vi "Init_Simulator(SubVI).vi"(10 "Enable 3D Visualization":bool, 11 "appended path":path) -> (0 "error out":errorcluster, 1 "robot body ref":refnum<k20>, 2 "starter kit differential steering frame":refnum<class "NI_Robotics_Differential Steering Frame.lvclass">, 3 "NI_Robotics_Starter Kit Host_Sim_2.0 out":refnum<class "NI_Robotics_Starter Kit Host_Sim_2.0.lvclass">, 5 "Current_Position":T1, 7 "map reference out":refnum<data-value>)   [LabVIEW 2017]
uses:
  Ctl/Current_Position.ctl
  <vilib>/robotics/Starter Kit/2.0/Sim Host Interface/NI_Robotics_Starter Kit Host_Sim_2.0.lvclass
  E:/PROGRAM FILES/National Instruments/LabVIEW 2017/vi.lib/robotics/Starter Kit/Host Interface/NI_Robotics_Starter Kit Host.lvclass
  <vilib>/robotics/Steering/Differential Steering Frame/NI_Robotics_Differential Steering Frame.lvclass
  <vilib>/robotics/Navigation/shared/WorldMap/OccupancyGridWorldMap/NI_Robotics_OccupancyGridWorldMap.lvclass
  <vilib>/robotics/Simulator/Interface/Simulator References/Get Robot Body Reference.vi
  GBL/GBL_variables.vi
  <vilib>/robotics/Simulator/NI_Robotics_Simulator.lvlib
  <vilib>/robotics/Starter Kit/2.0/NI_Robotics_Starter Kit Host_2.0.lvlib
  <resource>/objmgr/LVODE.rc
  <vilib>/robotics/Starter Kit/Host Interface/NI_Robotics_Starter Kit Host.lvclass
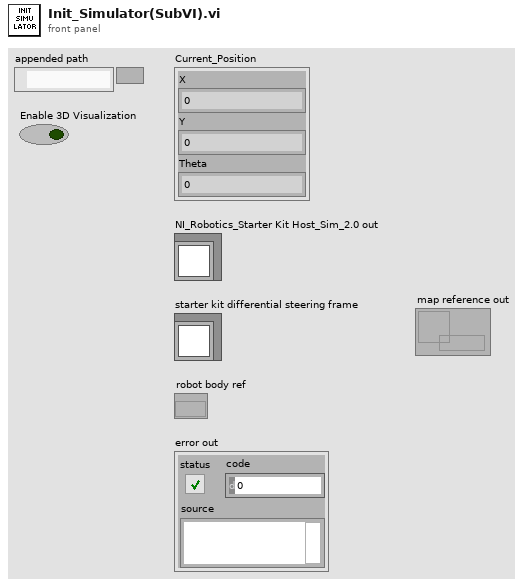
[diagram p1: front panel]
types:
  T1 = typedef "Current_Position.ctl" = cluster{"X":dbl, "Y":dbl, "Theta":dbl}
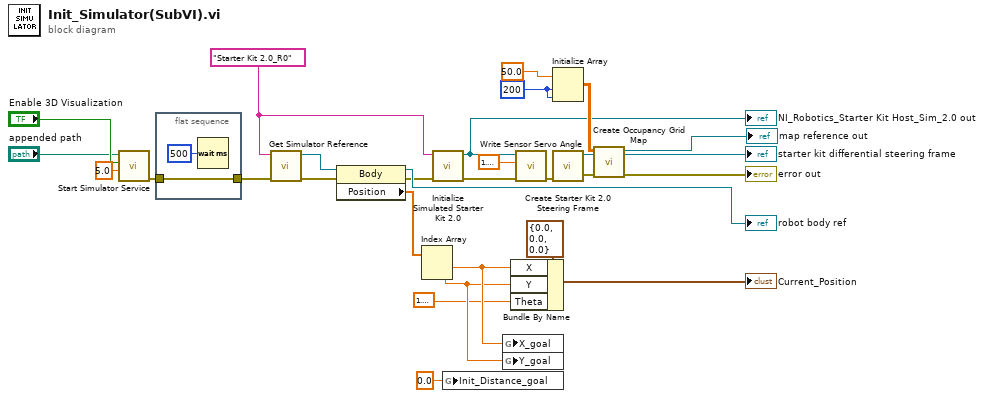
[diagram p0: block diagram]
diagram:
  w5 = 200 ("dimension size")
  w15 = "Starter Kit 2.0_R0" ("robot ID")
  n1 = call <vilib>:"Start Simulator Service.vi"("step size (ms)"=5.0, "enable 3D visualization (T)"="Enable 3D Visualization", "manifest file"="appended path") -> ("error out"=w20:errorcluster)  [unwired: 8 in]
  n2 = flat-sequence {
    tunnel: w20 -> [w30]
    tunnel: [w30] -> w21
    frame #0 {
      n3 = Wait (ms)(milliseconds to wait=u32 500) -> ()  [unwired: 1 out]
    }
  }
  n4 = call-poly <vilib>:"Get Simulator Reference.vi"("error in (no error)"=w21, "robot ID"=w15) -> ("error out"=w18:errorcluster, "robot body ref"=w16:refnum<k20>)  [unwired: 8 in]
  n5 = property class="Body"(reference=w16, error in=w18) -> (reference out=→"robot body ref":refnum<k20>, error out=w19:errorcluster, "Position"=w26:sgl[])
  n6 = Index Array(array=w26) -> (element #1=w11:sgl, element #2=w10:sgl)  [unwired: 2 in]
  n7 = call <vilib>:"Initialize Simulated Starter Kit 2.0.vi"("error in (no error)"=w19, "robot ID"=w15) -> ("error out"=w14:errorcluster, "simulated starter kit host 2.0 out"=w2:refnum<class "NI_Robotics_Starter Kit Host_Sim_2.0.lvclass">)  [unwired: 8 in]
  "NI_Robotics_Starter Kit Host_Sim_2.0 out" <- w2
  n8 = global write "GBL_variables.vi" "Init_Distance_goal"(0.0 ("Init_Distance_goal")) -> ()
  n9 = global write "GBL_variables.vi" "X_goal"(w11) -> ()
  n10 = global write "GBL_variables.vi" "Y_goal"(w10) -> ()
  n11 = Bundle By Name(cluster=T1 {"X"=0.0, "Y"=0.0, "Theta"=0.0} ("Current_Position"), "X"=w11, "Y"=w10, "Theta"=1.5707963267948966) -> (→"Current_Position":T1)
  n12 = call <vilib>:"Write Sensor Servo Angle.vi"("error in (no error)"=w14, "ccw servo angle (rad)"=1.5707963267948966, "starter kit host in"=w2) -> ("error out"=w3:errorcluster)  [unwired: 7 in, 1 out]
  n13 = Initialize Array(50.0 ("element"), w5, w5) -> (w4:dbl[][])
  n14 = call <vilib>:"Create Starter Kit 2.0 Steering Frame.vi"("error in (no error)"=w3) -> ("error out"=w24:errorcluster, "starter kit differential steering frame"=→"starter kit differential steering frame":refnum<class "NI_Robotics_Differential Steering Frame.lvclass">)  [unwired: 9 in]
  n15 = call <vilib>:"Create Occupancy Grid Map.vi"("error in (no error)"=w24, "occupancy grid"=w4) -> ("error out"=→"error out":errorcluster, "map reference out"=→"map reference out":refnum<data-value>)  [unwired: 8 in]
